vi "Read Radius (px).vi"(8 "error in (no error)":errorcluster, 11 "Geometric Figure in":refnum<class "UI Object.lvclass">) -> (0 "error out":errorcluster, 2 "Radius (px)":u16, 3 "Geometric Figure out":refnum<class "UI Object.lvclass">)   [LabVIEW 2016]
uses:
  UI Object.lvclass
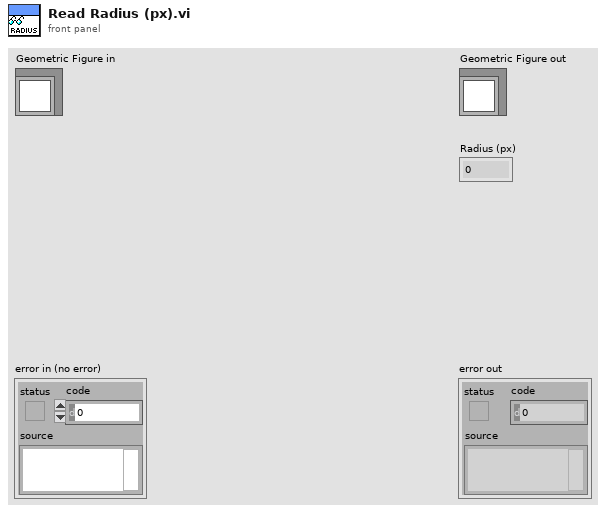
[diagram p1: front panel]
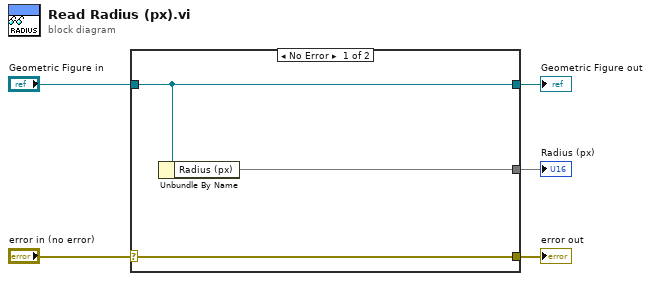
[diagram p0: block diagram]
diagram:
  n1 = case shown="No Error" "error in (no error)" {
    selector: "error in (no error)" -> [w8 w9]
    tunnel: [w8 w9] -> w4
    tunnel: [w7 w10] -> w2
    tunnel: "Geometric Figure in" -> [w7 w10]
    tunnel: [w6 _] -> w1
    frame No Error {
      n2 = Unbundle By Name(w7) -> ("Radius (px)"=w6)
    }
    frame Error {
    }
  }
  "error out" <- w4
  "Geometric Figure out" <- w2
  "Radius (px)" <- w1
